vi "CMN_modinfo.vi"(8 "error in (no error)":errorcluster, 10 "full":bool, 11 "caller path":path) -> (0 "error out":errorcluster, 2 "INFO":string)   [LabVIEW 2016]
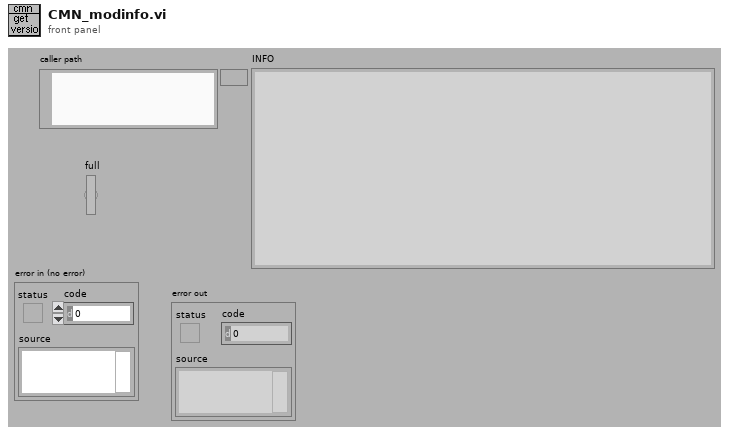
[diagram p1: front panel]
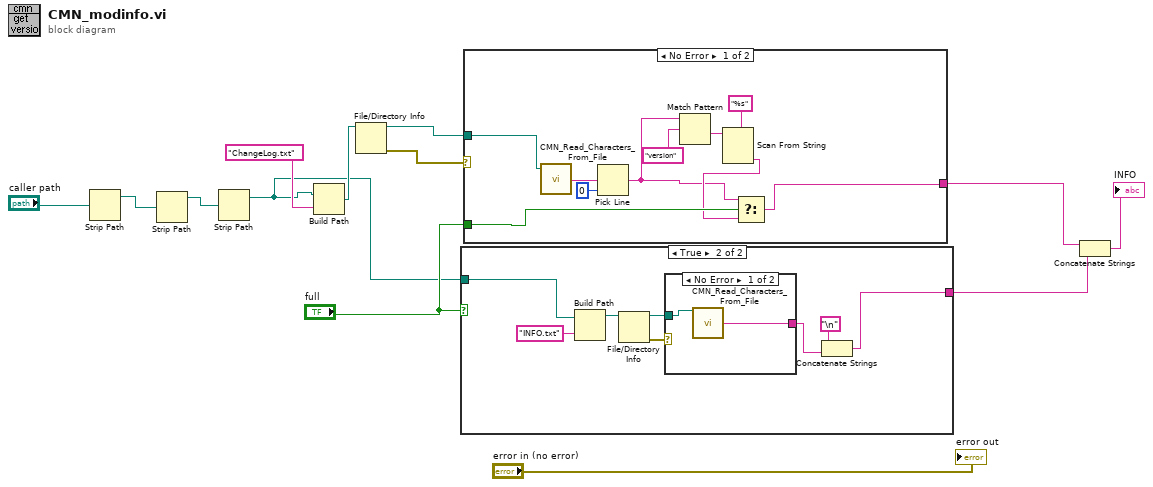
[diagram p0: block diagram]
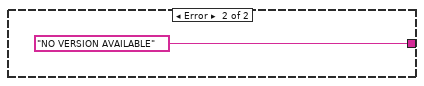
[diagram p2: hidden frame]
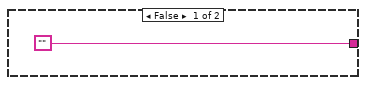
[diagram p3: hidden frame]
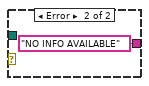
[diagram p4: hidden frame]
diagram:
  n1 = Strip Path(path="caller path") -> (stripped path=w12:path)  [unwired: 1 out]
  n2 = Strip Path(path=w12) -> (stripped path=w11:path)  [unwired: 1 out]
  n3 = Strip Path(path=w11) -> (stripped path=w2:path)  [unwired: 1 out]
  n4 = Build Path(base path=w2, name or relative path="ChangeLog.txt") -> (appended path=w9:path)
  n5 = File/Directory Info(path=w9) -> (path out=w1:path, error out=w3:errorcluster)  [unwired: 1 in, 5 out]
  n6 = case shown="True" "full" {
    tunnel: ["" w15] -> w4
    tunnel: w2 -> [_ w22]
    frame False {
    }
    frame True {
      n7 = Build Path(base path=w22, name or relative path="INFO.txt") -> (appended path=w20:path)
      n8 = File/Directory Info(path=w20) -> (path out=w18:path, error out=w19:errorcluster)  [unwired: 1 in, 5 out]
      n9 = case shown="No Error" w19 {
        tunnel: w18 -> [w24 _]
        tunnel: [w23 "NO INFO AVAILABLE" ("character string")] -> w16
        frame No Error {
          n10 = call "CMN_Read_Characters_From_File.vi"("file path"=w24) -> ("character string"=w23:string)  [unwired: 1 in, 7 out]
        }
        frame Error {
        }
      }
      n11 = Concatenate Strings("\n", w16) -> (w15:string)
    }
  }
  n12 = case shown="No Error" w3 {
    tunnel: w1 -> [w35 _]
    tunnel: [w26 "NO VERSION AVAILABLE" ("output string")] -> w5
    tunnel: "full" -> [w29 _]
    frame No Error {
      n13 = call "CMN_Read_Characters_From_File.vi"("file path"=w35) -> ("character string"=w34:string)  [unwired: 1 in, 7 out]
      n14 = Pick Line(multi-line string=w34, line index=0) -> (output string=w27:string)  [unwired: 1 out]
      n15 = Match Pattern(string=w27, regular expression="version") -> (after substring=w31:string)  [unwired: 4 out]
      n16 = Scan From String(format string="%s", input string=w31) -> (output 1=w28:string)  [unwired: 2 in, 4 out]
      n17 = Select(t=w27, s=w29, f=w28) -> (s? t:f=w26:string)
    }
    frame Error {
    }
  }
  n18 = Concatenate Strings(w5, w4) -> (→"INFO":string)
  "error out" <- "error in (no error)"
